vi "Send Response.vi"(8 "error in (no error)":errorcluster, 11 "Channel in":refnum<class "Channel.lvclass">) -> (0 "error out":errorcluster, 3 "Channel out":refnum<class "Channel.lvclass">)   [LabVIEW 2018, in "Channel.lvclass"]
uses:
  Channel.lvclass
  Channel.lvclass/Channel.ctl
  RxTx/RxTx.lvclass
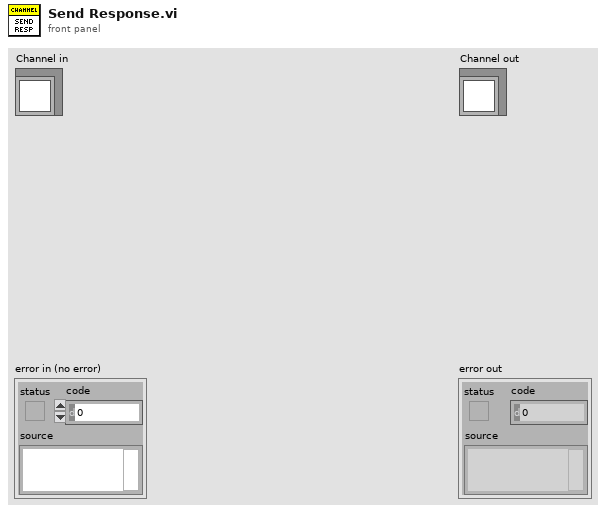
[diagram p1: front panel]
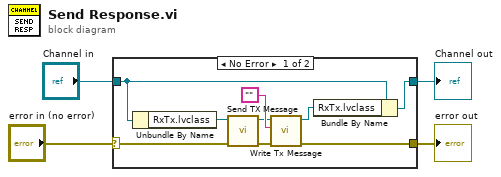
[diagram p0: block diagram]
diagram:
  n1 = case shown="No Error" "error in (no error)" {
    selector: "error in (no error)" -> [w12 w15]
    tunnel: [w11 w15] -> w3
    tunnel: [w6 w14] -> w1
    tunnel: "Channel in" -> [w7 w14]
    frame No Error {
      n2 = Unbundle By Name(w7) -> ("RxTx.lvclass"=w13:refnum<class "RxTx.lvclass">)
      n3 = call "Send TX Message.vi"("error in (no error)"=w12, "RxTx in"=w13) -> ("error out"=w10:errorcluster, "RxTx out"=w8:refnum<class "RxTx.lvclass">)  [unwired: 8 in]
      n4 = call "Write Tx Message.vi"("error in (no error)"=w10, "Tx Message"="" ("Response"), "RxTx in"=w8) -> ("error out"=w11:errorcluster, "RxTx out"=w5:refnum<class "RxTx.lvclass">)  [unwired: 7 in]
      n5 = Bundle By Name(cluster=w7, "RxTx.lvclass"=w5) -> (w6:refnum<class "Channel.lvclass">)
    }
    frame Error {
    }
  }
  "error out" <- w3
  "Channel out" <- w1
